vi "WS1050_51 VPI Header.vi"(0 "VPI Name":string[](array[string])=["All_Drivers OFF", "All Drivers ON", "All Drivers OFF2"], 5 "VPI_Cmd":string[](array[string])=["00", "3B", "00"], 7 "Cmin/Act":bool, 9 "WS1050/51":bool=TRUE, 11 "error in (no error)":errorcluster) -> (1 "VPI_1":string[](array[string]), 3 "VPI_2":string[](array[string]), 4 "VPI Header":string[](array[string]), 6 "VPI_3":string[](array[string]), 10 "Cmd_3":string[](array[string]), 12 "Cmd_1":string[](array[string]), 14 "Cmd_2":string[](array[string]), 15 "error out":errorcluster)   [LabVIEW 2012]
panel:
  in  "VPI_Cmd Cmin":string[](array[string])=["00", "00", "00"]
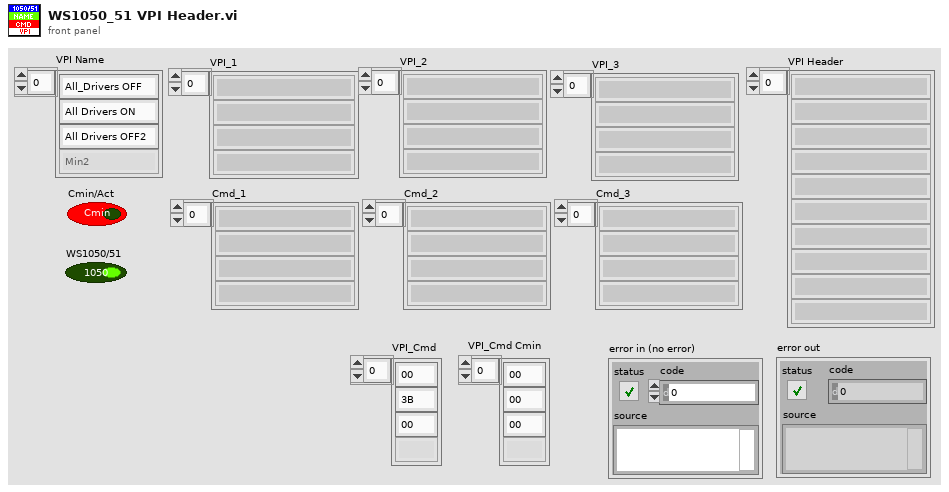
[diagram p1: front panel]
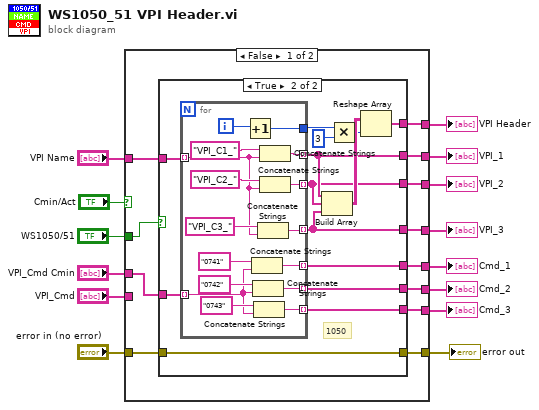
[diagram p0: block diagram]
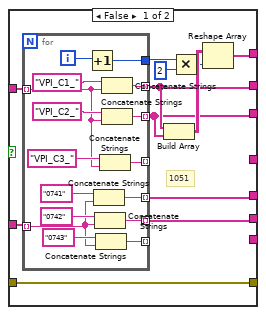
[diagram p2: hidden frame]
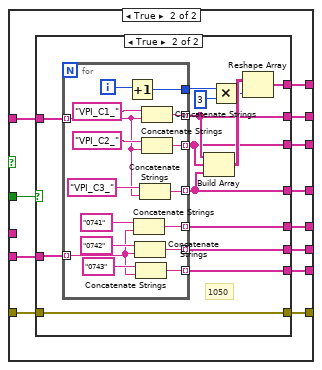
[diagram p3: hidden frame]
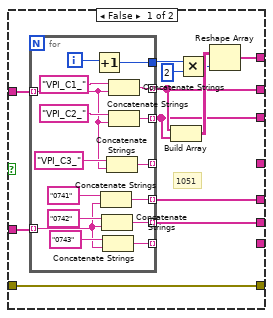
[diagram p4: hidden frame]
diagram:
  n1 = case shown="False" "Cmin/Act" {
    tunnel: "error in (no error)" -> [w16 w96]
    tunnel: [w15 w95] -> w13
    tunnel: "WS1050/51" -> [w17 w94]
    tunnel: "VPI_Cmd" -> [_ w93]
    tunnel: "VPI Name" -> [w18 w92]
    tunnel: [w26 w91] -> w9
    tunnel: [w25 w90] -> w8
    tunnel: [w24 w89] -> w7
    tunnel: [w23 w88] -> w6
    tunnel: [w22 w87] -> w5
    tunnel: [w21 w86] -> w4
    tunnel: [w20 w85] -> w3
    tunnel: "VPI_Cmd Cmin" -> [w19 _]
    frame False {
      n2 = case shown="True" w17 {
        tunnel: [w32 w64] -> w26
        tunnel: [w31 w63] -> w25
        tunnel: [w30 w62] -> w24
        tunnel: [_ w61] -> w23
        tunnel: [w29 w60] -> w22
        tunnel: [w28 w59] -> w21
        tunnel: [_ w58] -> w20
        tunnel: w19 -> [w34 w57]
        tunnel: w18 -> [w33 w56]
        tunnel: w16 -> [w27 w55]
        tunnel: [w27 w55] -> w15
        frame False {
          # "1051"
          n3 = for {
            tunnel: w33 -> [w39] mode=indexing
            tunnel: w34 -> [w45] mode=indexing
            tunnel: [w51] -> w31 mode=indexing
            tunnel: [w50] -> w30 mode=indexing
            tunnel: [w49] -> _ mode=indexing
            tunnel: [w44] -> w29 mode=indexing
            tunnel: [w43] -> w28 mode=indexing
            tunnel: [w42] -> _ mode=indexing
            tunnel: [w40] -> w37
            i -> [w41]
            n4 = Increment(x=w41) -> (x+1=w40:i32)
            n5 = Concatenate Strings("0741" ("string"), w45) -> (w44:string)
            n6 = Concatenate Strings("0742" ("string"), w45) -> (w43:string)
            n7 = Concatenate Strings("0743" ("string"), w45) -> (w42:string)
            n8 = Concatenate Strings("VPI_C3_" ("string"), w39) -> (w49:string)
            n9 = Concatenate Strings("VPI_C1_" ("string"), w39) -> (w51:string)
            n10 = Concatenate Strings("VPI_C2_" ("string"), w39) -> (w50:string)
          }
          n11 = Build Array(w31, w30) -> (w38:string[][])
          n12 = Multiply(x=w37, y=2) -> (x*y=w36:i32)
          n13 = Reshape Array(w38, w36) -> (w32:string[])
        }
        frame True {
          # "1050"
          n14 = for {
            tunnel: w56 -> [w69] mode=indexing
            tunnel: w57 -> [w75] mode=indexing
            tunnel: [w81] -> w63 mode=indexing
            tunnel: [w80] -> w62 mode=indexing
            tunnel: [w79] -> w61 mode=indexing
            tunnel: [w74] -> w60 mode=indexing
            tunnel: [w73] -> w59 mode=indexing
            tunnel: [w72] -> w58 mode=indexing
            tunnel: [w70] -> w67
            i -> [w71]
            n15 = Increment(x=w71) -> (x+1=w70:i32)
            n16 = Concatenate Strings("0741" ("string"), w75) -> (w74:string)
            n17 = Concatenate Strings("0742" ("string"), w75) -> (w73:string)
            n18 = Concatenate Strings("0743" ("string"), w75) -> (w72:string)
            n19 = Concatenate Strings("VPI_C3_" ("string"), w69) -> (w79:string)
            n20 = Concatenate Strings("VPI_C1_" ("string"), w69) -> (w81:string)
            n21 = Concatenate Strings("VPI_C2_" ("string"), w69) -> (w80:string)
          }
          n22 = Build Array(w63, w62, w61) -> (w68:string[][])
          n23 = Multiply(x=w67, y=3) -> (x*y=w66:i32)
          n24 = Reshape Array(w68, w66) -> (w64:string[])
        }
      }
    }
    frame True {
      n25 = case shown="True" w94 {
        tunnel: w96 -> [w97 w134]
        tunnel: [w97 w134] -> w95
        tunnel: w93 -> [w103 w133]
        tunnel: w92 -> [w104 w132]
        tunnel: [w102 w131] -> w91
        tunnel: [w101 w130] -> w90
        tunnel: [w100 w129] -> w89
        tunnel: [_ w128] -> w88
        tunnel: [w99 w127] -> w87
        tunnel: [w98 w126] -> w86
        tunnel: [_ w125] -> w85
        frame False {
          # "1051"
          n26 = for {
            tunnel: w104 -> [w109] mode=indexing
            tunnel: w103 -> [w115] mode=indexing
            tunnel: [w121] -> w101 mode=indexing
            tunnel: [w120] -> w100 mode=indexing
            tunnel: [w119] -> _ mode=indexing
            tunnel: [w114] -> w99 mode=indexing
            tunnel: [w113] -> w98 mode=indexing
            tunnel: [w112] -> _ mode=indexing
            tunnel: [w110] -> w107
            i -> [w111]
            n27 = Increment(x=w111) -> (x+1=w110:i32)
            n28 = Concatenate Strings("0741" ("string"), w115) -> (w114:string)
            n29 = Concatenate Strings("0742" ("string"), w115) -> (w113:string)
            n30 = Concatenate Strings("0743" ("string"), w115) -> (w112:string)
            n31 = Concatenate Strings("VPI_C3_" ("string"), w109) -> (w119:string)
            n32 = Concatenate Strings("VPI_C1_" ("string"), w109) -> (w121:string)
            n33 = Concatenate Strings("VPI_C2_" ("string"), w109) -> (w120:string)
          }
          n34 = Build Array(w101, w100) -> (w108:string[][])
          n35 = Multiply(x=w107, y=2) -> (x*y=w106:i32)
          n36 = Reshape Array(w108, w106) -> (w102:string[])
        }
        frame True {
          # "1050"
          n37 = for {
            tunnel: w132 -> [w139] mode=indexing
            tunnel: w133 -> [w145] mode=indexing
            tunnel: [w151] -> w130 mode=indexing
            tunnel: [w150] -> w129 mode=indexing
            tunnel: [w149] -> w128 mode=indexing
            tunnel: [w144] -> w127 mode=indexing
            tunnel: [w143] -> w126 mode=indexing
            tunnel: [w142] -> w125 mode=indexing
            tunnel: [w140] -> w137
            i -> [w141]
            n38 = Increment(x=w141) -> (x+1=w140:i32)
            n39 = Concatenate Strings("0741" ("string"), w145) -> (w144:string)
            n40 = Concatenate Strings("0742" ("string"), w145) -> (w143:string)
            n41 = Concatenate Strings("0743" ("string"), w145) -> (w142:string)
            n42 = Concatenate Strings("VPI_C3_" ("string"), w139) -> (w149:string)
            n43 = Concatenate Strings("VPI_C1_" ("string"), w139) -> (w151:string)
            n44 = Concatenate Strings("VPI_C2_" ("string"), w139) -> (w150:string)
          }
          n45 = Build Array(w130, w129, w128) -> (w138:string[][])
          n46 = Multiply(x=w137, y=3) -> (x*y=w136:i32)
          n47 = Reshape Array(w138, w136) -> (w131:string[])
        }
      }
    }
  }
  "error out" <- w13
  "VPI_1" <- w8
  "VPI_2" <- w7
  "VPI_3" <- w6
  "Cmd_1" <- w5
  "Cmd_2" <- w4
  "Cmd_3" <- w3
  "VPI Header" <- w9
